vi "Initialize Device Core.vi"(8 "error in (no error)":errorcluster, 9 "Reset (F)":bool, 10 "Resource Name":string, 11 "CS++IEFWerner in":refnum<class "CS++IEFWerner.lvclass">) -> (0 "error out":errorcluster, 3 "CS++IEFWerner out":refnum<class "CS++IEFWerner.lvclass">)   [LabVIEW 2015, in "CS++IEFWerner.lvlib" / "CS++IEFWerner.lvclass"]
doc: "Initialize device driver."
uses:
  CS++IEFWerner.lvclass
  CSPP_Core/Classes/CS++ProcessVariables/ProcessVariable/PV.lvclass
  CS++IEFWerner.lvclass/CS++IEFWerner.ctl
  CSPP_Core/Classes/CS++ProcessVariables/ProcessVariable/PV.lvclass/PV.ctl
  CSPP_Core/Classes/CS++ProcessVariables/ProcessVariable/Write Data.vi
  CSPP_Core/Classes/CS++ProcessVariables/ProcessVariable/Write Timestamp.vi
  CSPP_Core/Classes/CS++ProcessVariables/ProcessVariable/Write Quality.vi
  CSPP_Core/Classes/CS++ProcessVariables/ProcessVariable/Write status.vi
  CSPP_DeviceBase/CS++Motor/CS++Motor.lvclass
  CSPP_Core/Classes/CS++ProcessVariables/PVConnection/PVConnection.lvclass
  instr.lib/IEF-pac/IEF Werner.lvlib
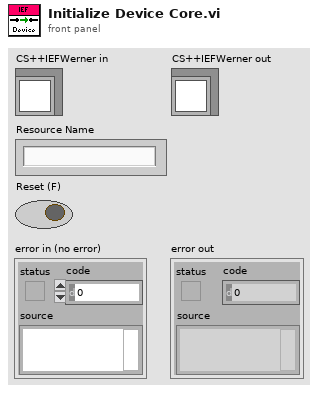
[diagram p1: front panel]
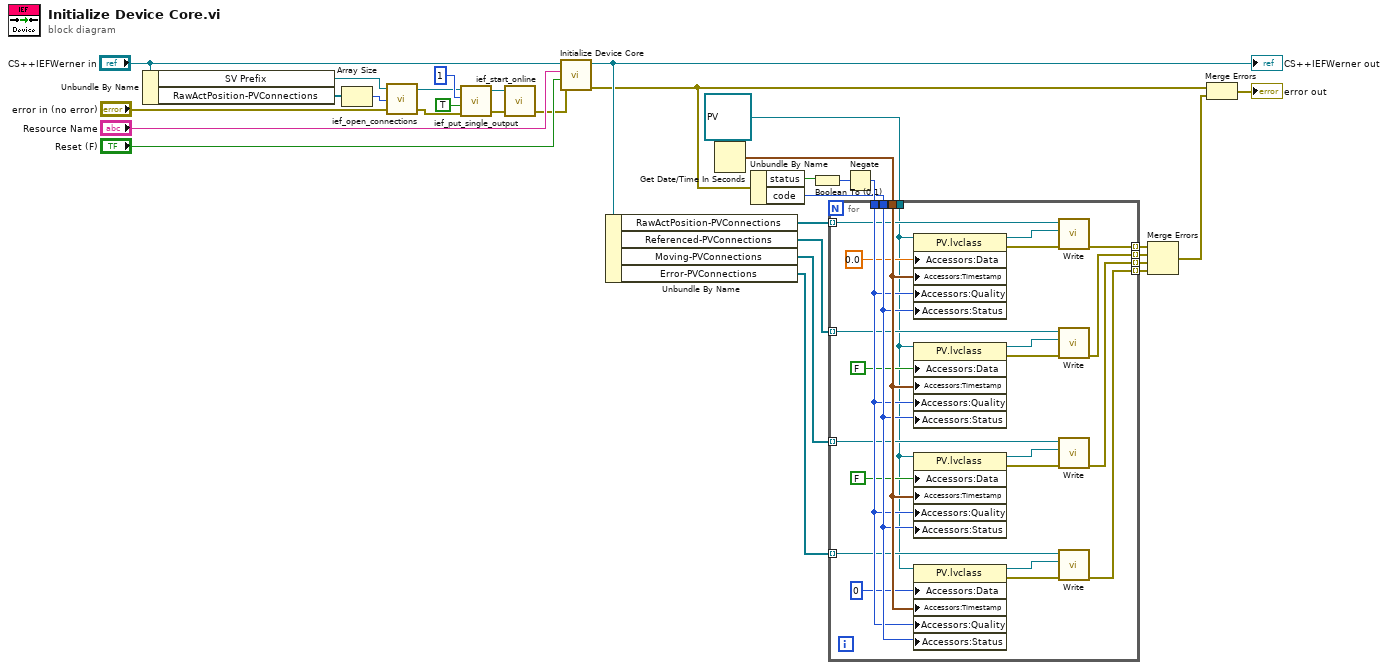
[diagram p0: block diagram]
diagram:
  n1 = Unbundle By Name("CS++IEFWerner in") -> ("SV Prefix"=w8:refnum<k21>, "RawActPosition-PVConnections"=w10:refnum<class "PVConnection.lvclass">[])
  n2 = Array Size(array=w10) -> (size(s)=w9:i32)
  n3 = call "ief_open_connections.vi"("error in (no error)"="error in (no error)", "NumberOfAxes"=w9, "Tagprefix in"=w8) -> ("error out (no error)"=w3:errorcluster, "Tagprefix out"=w2:refnum<k21>)  [unwired: 1 in]
  n4 = call "ief_put_single_output.vi"("error in (no error)"=w3, "Single Output State"=TRUE, "Single Output Number"=u16 1, "Tagprefix in"=w2) -> ("error out (no error)"=w6:errorcluster, "Tagprefix out"=w7:refnum<k21>)  [unwired: 1 out]
  n5 = call "ief_start_online.vi"("Tagprefix in"=w7, "error in (no error)"=w6) -> ("error out (no error)"=w1:errorcluster)  [unwired: 2 out]
  n6 = call-parent "Initialize Device Core.vi"("error in (no error)"=w1, "Reset (F)"="Reset (F)", "Resource Name"="Resource Name", "CS++Motor in"="CS++IEFWerner in") -> ("error out"=w13:errorcluster, "CS++Motor out"=w14:refnum<class "CS++IEFWerner.lvclass">)  [unwired: 6 in]
  "CS++IEFWerner out" <- w14
  n7 = Unbundle By Name(w14) -> ("RawActPosition-PVConnections"=w26:refnum<class "PVConnection.lvclass">[], "Referenced-PVConnections"=w27:refnum<class "PVConnection.lvclass">[], "Moving-PVConnections"=w28:refnum<class "PVConnection.lvclass">[], "Error-PVConnections"=w29:refnum<class "PVConnection.lvclass">[])
  n8 = Get Date/Time In Seconds() -> (seconds since 1Jan1904=w21:timestamp)
  n9 = Unbundle By Name(w13) -> ("status"=w19:bool, "code"=w22:i32)
  n10 = Boolean To (0,1)(Boolean=w19) -> (0, 1=w16:i16)
  n11 = Negate(x=w16) -> (-x=w23:i16)
  n12 = for {
    tunnel: [w52] -> w17 mode=indexing
    tunnel: [w51] -> w18 mode=indexing
    tunnel: refnum<class "PV.lvclass"> refnum ("PV") -> [w34]
    tunnel: w21 -> [w46]
    tunnel: w22 -> [w45]
    tunnel: w23 -> [w44]
    tunnel: [w43] -> w24 mode=indexing
    tunnel: [w42] -> w25 mode=indexing
    tunnel: w26 -> [w41] mode=indexing
    tunnel: w27 -> [w40] mode=indexing
    tunnel: w28 -> [w39] mode=indexing
    tunnel: w29 -> [w38] mode=indexing
    n13 = property class="PV.lvclass"(reference=w34, "Accessors:Data"=0.0, "Accessors:Timestamp"=w46, "Accessors:Quality"=w44, "Accessors:Status"=w45) -> (reference out=w56:refnum<class "PV.lvclass">, error out=w55:errorcluster)  [unwired: 1 in]
    n14 = property class="PV.lvclass"(reference=w34, "Accessors:Data"=FALSE, "Accessors:Timestamp"=w46, "Accessors:Quality"=w44, "Accessors:Status"=w45) -> (reference out=w54:refnum<class "PV.lvclass">, error out=w53:errorcluster)  [unwired: 1 in]
    n15 = property class="PV.lvclass"(reference=w34, "Accessors:Data"=FALSE, "Accessors:Timestamp"=w46, "Accessors:Quality"=w44, "Accessors:Status"=w45) -> (reference out=w49:refnum<class "PV.lvclass">, error out=w50:errorcluster)  [unwired: 1 in]
    n16 = property class="PV.lvclass"(reference=w34, "Accessors:Data"=i8 0, "Accessors:Timestamp"=w46, "Accessors:Quality"=w44, "Accessors:Status"=w45) -> (reference out=w47:refnum<class "PV.lvclass">, error out=w48:errorcluster)  [unwired: 1 in]
    n17 = call "Write.vi"("error in (no error)"=w55, "PV"=w56, "PVConnection in"=w41) -> ("error out"=w52:errorcluster)  [unwired: 7 in, 1 out]
    n18 = call "Write.vi"("error in (no error)"=w53, "PV"=w54, "PVConnection in"=w40) -> ("error out"=w51:errorcluster)  [unwired: 7 in, 1 out]
    n19 = call "Write.vi"("error in (no error)"=w50, "PV"=w49, "PVConnection in"=w39) -> ("error out"=w43:errorcluster)  [unwired: 7 in, 1 out]
    n20 = call "Write.vi"("error in (no error)"=w48, "PV"=w47, "PVConnection in"=w38) -> ("error out"=w42:errorcluster)  [unwired: 7 in, 1 out]
  }
  n21 = Merge Errors(w17, w18, w24, w25) -> (w30:errorcluster)
  n22 = Merge Errors(w13, w30) -> (→"error out":errorcluster)
